vi "controlRealtimeInputStepsPerPulse.vi"(7 "Set":bool, 8 "error in":errorcluster, 9 "Steps in":i32, 10 "axis in":u8, 11 "connection ID":refnum<k5>) -> (0 "error out":errorcluster, 1 "Steps out":i32, 2 "axis out":u8, 3 "connection ID":refnum<k5>)   [LabVIEW 2016]
panel:
  in  "Set Command":string="com.attocube.amc.rtin.setRealTimeInStepsPerPulse"
  in  "Get Command":string="com.attocube.amc.rtin.getRealTimeInStepsPerPulse"
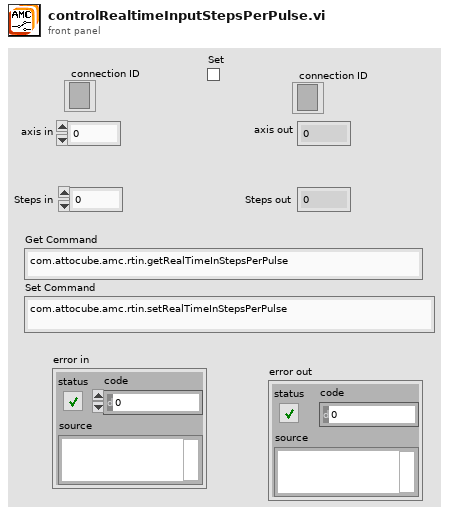
[diagram p1: front panel]
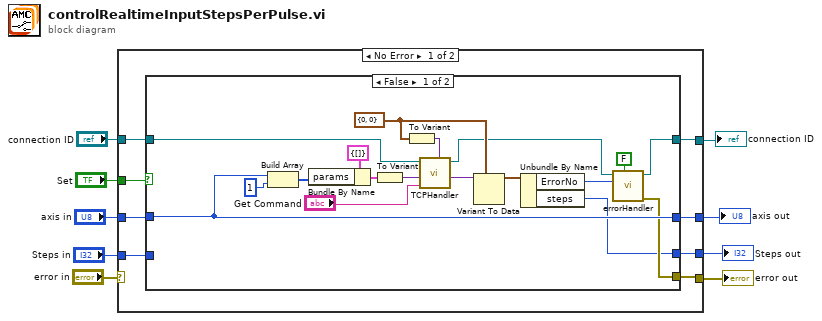
[diagram p0: block diagram]
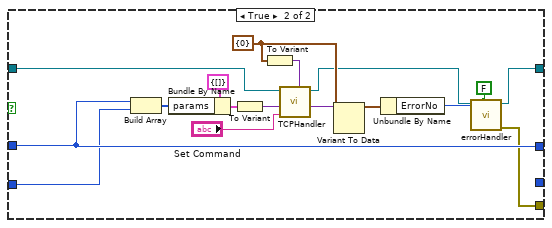
[diagram p2: hidden frame]
diagram:
  n1 = case shown="No Error" "error in" {
    selector: "error in" -> [_ w55]
    tunnel: "axis in" -> [w15 w54]
    tunnel: [w10 w55] -> w8
    tunnel: [w12 w54] -> w7
    tunnel: "Set" -> [w16 _]
    tunnel: [w13 w53] -> w5
    tunnel: "connection ID" -> [w17 w53]
    tunnel: "Steps in" -> [w14 w56]
    tunnel: [w11 w56] -> w2
    frame No Error {
      n2 = case shown="False" w16 {
        tunnel: [w18 w36] -> w13
        tunnel: w17 -> [w25 w47]
        tunnel: w15 -> [w27 w45]
        tunnel: [w27 w45] -> w12
        tunnel: [w26 w42] -> w10
        tunnel: [w22 _] -> w11
        tunnel: w14 -> [_ w39]
        frame False {
          w23 = cluster{"ErrorNo":i16, "steps":i64} {"ErrorNo"=0, "steps"=0} ("input cluster")
          n3 = Build Array(w27, u8 1 ("element")) -> (w31:u8[])
          n4 = Bundle By Name(cluster=cluster{"params":i16[]} {"params"=[]} ("input cluster"), "params"=w31) -> (w32:cluster{"params":i16[]})
          n5 = To Variant(anything=w32) -> (Variant=w33:variant)
          n6 = To Variant(anything=w23) -> (Variant=w24:variant)
          n7 = call "TCPHandler.vi"("result Types"=w24, "method"="Get Command", "params"=w33, "connection ID"=w25) -> ("result"=w29:variant, "connection ID"=w19:refnum<k5>)  [unwired: 5 in, 1 out]
          n8 = Variant To Data(type=w23, Variant=w29) -> (data=w34:cluster{"ErrorNo":i16, "steps":i64})  [unwired: 1 in, 1 out]
          n9 = Unbundle By Name(w34) -> ("ErrorNo"=w35:i16, "steps"=w22:i64)
          n10 = call "errorHandler.vi"("show popup"=FALSE, "error number"=w35, "connection ID"=w19) -> ("error out"=w26:errorcluster, "connection ID"=w18:refnum<k5>)  [unwired: 7 in]
        }
        frame True {
          w40 = cluster{"ErrorNo":i16} {"ErrorNo"=0} ("input cluster")
          n11 = Build Array(w45, w39) -> (w49:i32[])
          n12 = Bundle By Name(cluster=cluster{"params":i64[]} {"params"=[]} ("input cluster"), "params"=w49) -> (w48:cluster{"params":i64[]})
          n13 = To Variant(anything=w48) -> (Variant=w46:variant)
          n14 = To Variant(anything=w40) -> (Variant=w41:variant)
          n15 = call "TCPHandler.vi"("result Types"=w41, "method"="Set Command", "params"=w46, "connection ID"=w47) -> ("result"=w51:variant, "connection ID"=w37:refnum<k5>)  [unwired: 5 in, 1 out]
          n16 = Variant To Data(type=w40, Variant=w51) -> (data=w44:cluster{"ErrorNo":i16})  [unwired: 1 in, 1 out]
          n17 = Unbundle By Name(w44) -> ("ErrorNo"=w43:i16)
          n18 = call "errorHandler.vi"("show popup"=FALSE, "error number"=w43, "connection ID"=w37) -> ("error out"=w42:errorcluster, "connection ID"=w36:refnum<k5>)  [unwired: 7 in]
        }
      }
    }
    frame Error {
    }
  }
  "error out" <- w8
  "axis out" <- w7
  "connection ID" <- w5
  "Steps out" <- w2
